vi "checksum.vi"(8 "error in (no error)":errorcluster, 10 "input":string, 11 "CEG4500 in":refnum<class "CEG4500.lvclass">) -> (0 "error out":errorcluster, 2 "output":string, 3 "CEG4500 out":refnum<class "CEG4500.lvclass">)   [LabVIEW 2013, in "CEG4500.lvclass"]
uses:
  CEG4500.lvclass
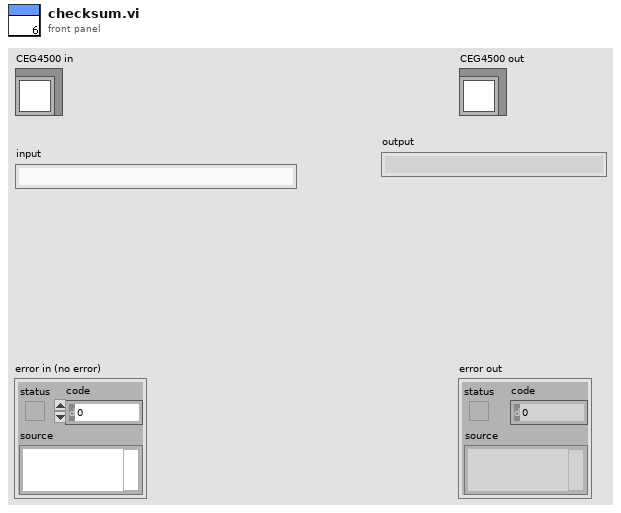
[diagram p1: front panel]
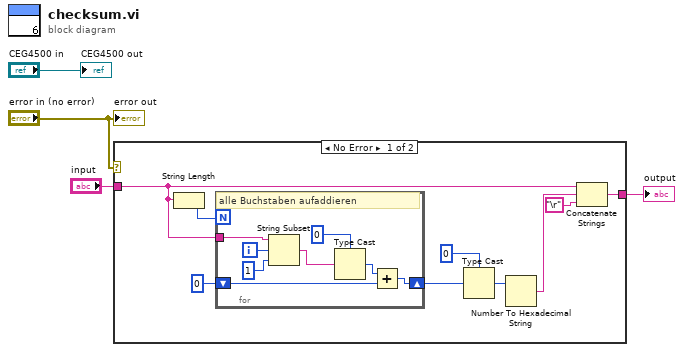
[diagram p0: block diagram]
diagram:
  n1 = case shown="No Error" "error in (no error)" {
    tunnel: "input" -> [w5 w22]
    tunnel: [w6 w22] -> w3
    frame No Error {
      n2 = String Length(string=w5) -> (length=w7:i32)
      n3 = for {
        N: w7 -> [_]
        shift-right: [w16] -> w9
        shift-left: 0 -> [w17]
        tunnel: w5 -> [w14]
        i -> [w15]
        # "alle Buchstaben aufaddieren"
        n4 = String Subset(string=w14, offset (0)=w15, length (rest)=1 ("length (rest)")) -> (substring=w19:string)
        n5 = Type Cast(type=0, x=w19) -> (*(type *) &x=w18:i32)
        n6 = Add(x=w18, y=w17) -> (x+y=w16:i32)
      }
      n7 = Type Cast(type=i8 0 ("unit (none)"), x=w9) -> (*(type *) &x=w12:i8)
      n8 = Number To Hexadecimal String(2:w12) -> (0:w10:string)  [unwired: 1 in]
      n9 = Concatenate Strings(w5, w10, "\r") -> (w6:string)
    }
    frame Error {
    }
  }
  "output" <- w3
  "error out" <- "error in (no error)"
  "CEG4500 out" <- "CEG4500 in"
